vi "Calculate Pixel Reciprocals.vi"(9 "Bottom":T2, 10 "Middle":T2, 11 "Top":T2) -> (3 "Columns Pixels Per Row":T1)   [LabVIEW 2022 SP3, in "Raster.lvlib"]
uses:
  Raster.lvlib
  Point 2D.ctl
  Reciprocals.ctl
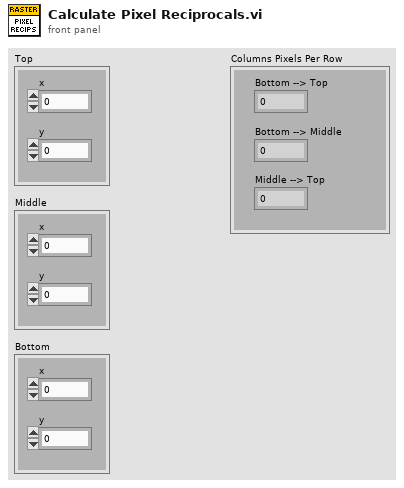
[diagram p1: front panel]
types:
  T1 = typedef "Raster.lvlib/Reciprocals.ctl" = cluster{"Bottom --> Top":sgl, "Bottom --> Middle":sgl, "Middle --> Top":sgl}
  T2 = typedef "Raster.lvlib/Point 2D.ctl" = cluster{"x":i32, "y":i32}
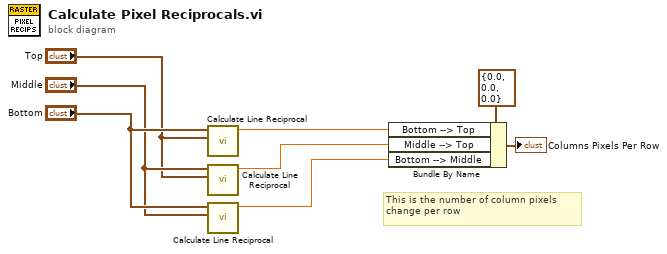
[diagram p0: block diagram]
diagram:
  # "This is the number of column pixels change per row"
  n1 = call "Calculate Line Reciprocal.vi"("P2"="Top", "P1"="Bottom") -> ("Column Pixels Per Row"=w4:sgl)  [unwired: 9 in]
  n2 = call "Calculate Line Reciprocal.vi"("P2"="Top", "P1"="Middle") -> ("Column Pixels Per Row"=w5:sgl)  [unwired: 9 in]
  n3 = call "Calculate Line Reciprocal.vi"("P2"="Middle", "P1"="Bottom") -> ("Column Pixels Per Row"=w6:sgl)  [unwired: 9 in]
  n4 = Bundle By Name(cluster=T1 {"Bottom --> Top"=0.0, "Bottom --> Middle"=0.0, "Middle --> Top"=0.0} ("Reciprocals"), "Bottom --> Top"=w4, "Middle --> Top"=w5, "Bottom --> Middle"=w6) -> (→"Columns Pixels Per Row":T1)
